vi "Call (async).vi"   [LabVIEW 2020, in "wamplv.lvlib" / "WAMP Client.lvclass"]
uses:
  WAMP Client.lvclass
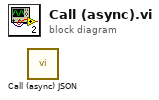
[diagram p0: block diagram]
diagram:
  n1 = call "Call (async) JSON.vi"() -> ()  [unwired: 9 in, 3 out]
